vi "tlc_Move Cue.vi"(7 "Cue Operation":enum16{"Move Cue Up", "Move Cue Down"}(ring), 8 "error in (no error)":errorcluster, 10 "Selected Cue":i32) -> (0 "error out":errorcluster)   [LabVIEW 2018]
doc: "This VI will move a cue up or down in the cue list. This VI will rearrange a Cue by simply swapping cues in the Cue module."
uses:
  Modules/Cue/tlc_Cue_Information Command.ctl
  Controls/tlc_User Interface Data Type.ctl
panel:
  # "Input"
  # "Output"
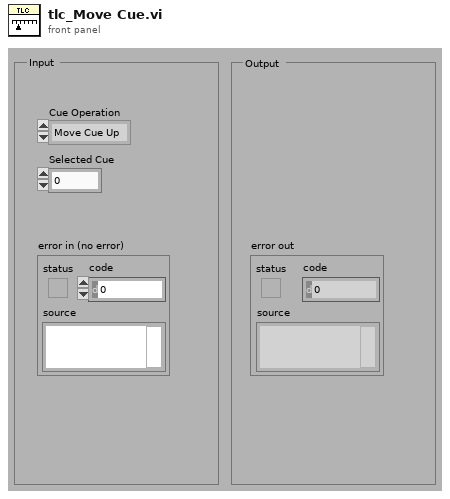
[diagram p1: front panel]
types:
  T1 = typedef "tlc_Cue_Information Command.ctl" = enum16{"Add Cue", "Delete Cue", "Get Cue Values", "Set Cue Values", "Swap", "Get Number of Cues", "Initialize", "Get Empty Cue"}
  T2 = typedef "tlc_User Interface Data Type.ctl" = enum16{"Initialize", "Initialize Front Panel", "Update Front Panel Channels", "Select Cue in Cue List", "Enable/Disable Front Panel Controls", "Update Cue List", "Stop"}
  T3 = typedef "tlc_Cue_Information.ctl" = cluster{"Cue Name":string, "Wait Time (s)":u32, "Fade Time (s)":u32, "Follow Time (s)":u32, "Channels":T4[][]}
  T4 = typedef "channel.ctl" = cluster{"Intensity":dbl, " Color":u32, "Channel":i32}
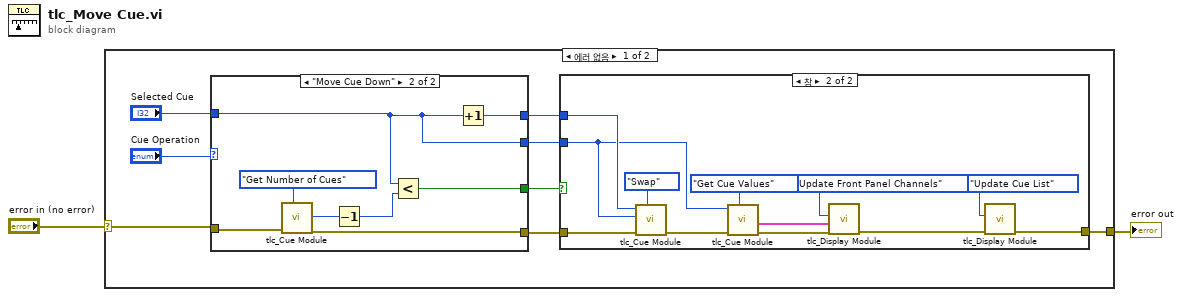
[diagram p0: block diagram]
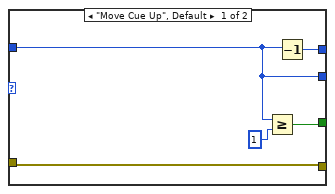
[diagram p2: hidden frame]
diagram:
  n1 = case shown="에러 없음" "error in (no error)" {
    selector: "error in (no error)" -> [w5 w37]
    tunnel: [w3 w37] -> w1
    frame No Error {
      n2 = case shown="\"Move Cue Down\"" "Cue Operation" {
        tunnel: "Selected Cue" -> [w11 w19]
        tunnel: [w15 w21] -> w8
        tunnel: [w12 w20] -> w7
        tunnel: [w11 w19] -> w6
        tunnel: w5 -> [w13 w18]
        tunnel: [w13 w17] -> w4
        frame "Move Cue Up", Default {
          n3 = Greater Or Equal?(x=w11, y=1) -> (x >= y?=w15:bool)
          n4 = Decrement(x=w11) -> (x-1=w12:i32)
        }
        frame "Move Cue Down" {
          n5 = call "tlc_Cue Module.vi"("Command"=tlc_Cue_Information_Command."Get Number of Cues" ("Enum"), "error in (no error)"=w18) -> ("error out"=w17:errorcluster, "Number of Cues"=w23:i32)  [unwired: 6 in, 1 out]
          n6 = Decrement(x=w23) -> (x-1=w22:i32)
          n7 = Less?(x=w19, y=w22) -> (x < y?=w21:bool)
          n8 = Increment(x=w19) -> (x+1=w20:i32)
        }
      }
      n9 = case shown="참" w8 {
        tunnel: w7 -> [_ w35]
        tunnel: w6 -> [_ w33]
        tunnel: w4 -> [w24 w36]
        tunnel: [w24 w25] -> w3
        frame False {
        }
        frame True {
          n10 = call "tlc_Cue Module.vi"("Command"=tlc_Cue_Information_Command."Swap" ("Enum"), "error in (no error)"=w36, "Swap Index"=w33, "Cue Index"=w35) -> ("error out"=w34:errorcluster)  [unwired: 4 in, 2 out]
          n11 = call "tlc_Cue Module.vi"("Command"=tlc_Cue_Information_Command."Get Cue Values" ("Enum"), "error in (no error)"=w34, "Cue Index"=w33) -> ("error out"=w32:errorcluster, "Cue Output"=w28:T3)  [unwired: 5 in, 1 out]
          n12 = call "tlc_Display Module.vi"("error in (no error)"=w32, "Data"=w28, "Data Type"=tlc_User_Interface_Data_Type."Update Front Panel Channels") -> ("error out"=w27:errorcluster)  [unwired: 8 in]
          n13 = call "tlc_Display Module.vi"("error in (no error)"=w27, "Data Type"=tlc_User_Interface_Data_Type."Update Cue List") -> ("error out"=w25:errorcluster)  [unwired: 9 in]
        }
      }
    }
    frame Error {
    }
  }
  "error out" <- w1
